vi "Differential Drive Chassis to Wheel Speed.vi"(9 "trackWidth":dbl, 10 "omega":dbl, 11 "vx":dbl) -> (2 "right":dbl, 3 "left":dbl)   [LabVIEW 2019]
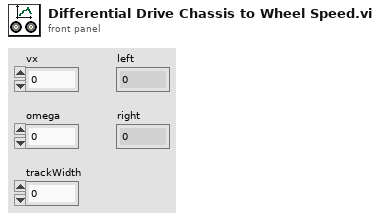
[diagram p1: front panel]
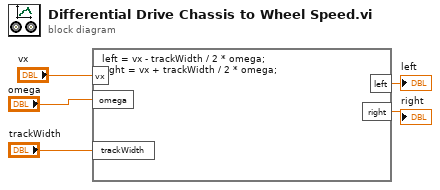
[diagram p0: block diagram]
diagram:
  n1 = formula code="left = vx - trackWidth / 2 * omega;\nright = vx + trackWidth / 2 * omega;"("vx"="vx", "omega"="omega", "trackWidth"="trackWidth") -> ("left"=→"left":dbl, "right"=→"right":dbl)
